vi "reset_channel.vi"(8 "error in (no error)":errorcluster, 10 "channel":T1=enum."1", 11 "Motech-pps-1200 in":refnum<class "Motech-pps-1200.lvclass">) -> (0 "error out":errorcluster, 3 "Motech-pps-1200 out":refnum<class "Motech-pps-1200.lvclass">)   [LabVIEW 2017, in "Motech-pps-1200.lvclass"]
uses:
  Motech-pps-1200.lvclass
  subVI/motech_power_supply/types/motech_set_value_cluster.ctl
  subVI/motech_power_supply/types/channels_enum.ctl
panel:
  in  "motech_set_value":T2={"voltage"=0.0, "current"=0.01, "channel"=enum."1"}
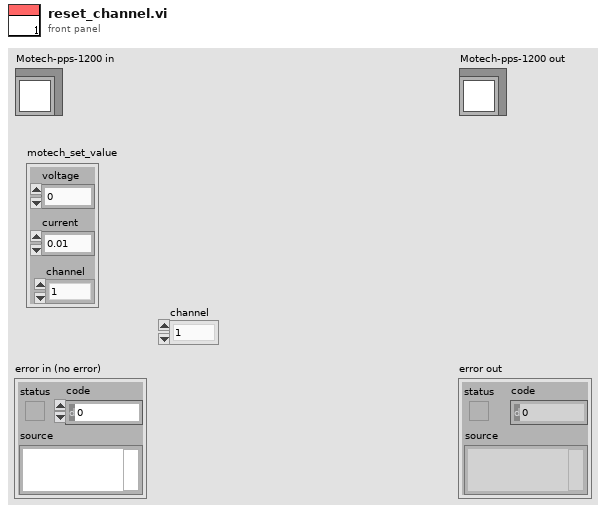
[diagram p1: front panel]
types:
  T1 = typedef "channels_enum.ctl" = enum16{"0", "1", "2"}
  T2 = typedef "motech_set_value_cluster.ctl" = cluster{"voltage":dbl, "current":dbl, "channel":T1}
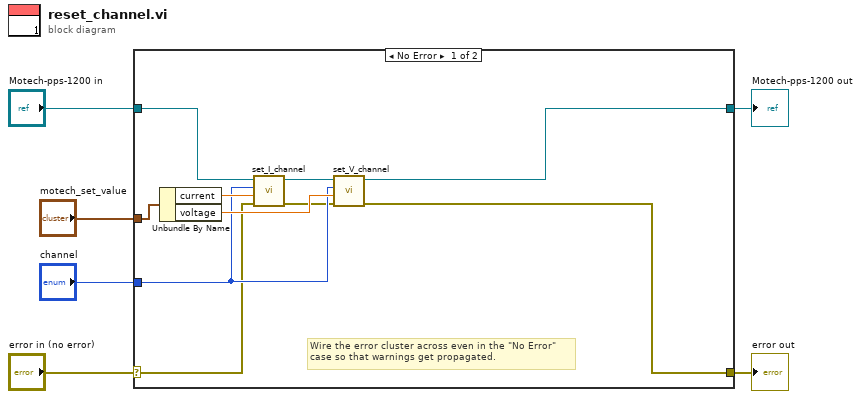
[diagram p0: block diagram]
diagram:
  n1 = case shown="No Error" "error in (no error)" {
    selector: "error in (no error)" -> [w9 w18]
    tunnel: [w7 w18] -> w5
    tunnel: [w14 w17] -> w3
    tunnel: "Motech-pps-1200 in" -> [w16 w17]
    tunnel: "motech_set_value" -> [w13 _]
    tunnel: "channel" -> [w10 _]
    frame No Error {
      # "Wire the error cluster across even in the \"No Error\"\ncase so that warnings get propagated."
      n2 = Unbundle By Name(w13) -> ("current"=w12:dbl, "voltage"=w11:dbl)
      n3 = call-dynamic "set_I_channel.vi"("error in (no error)"=w9, "current"=w12, "channel"=w10, "Motech-pps-1200 in"=w16) -> ("error out"=w8:errorcluster, "Motech-pps-1200 out"=w15:refnum<class "Motech-pps-1200.lvclass">)  [unwired: 6 in]
      n4 = call-dynamic "set_V_channel.vi"("error in (no error)"=w8, "voltage"=w11, "channel"=w10, "Motech-pps-1200 in"=w15) -> ("error out"=w7:errorcluster, "Motech-pps-1200 out"=w14:refnum<class "Motech-pps-1200.lvclass">)  [unwired: 6 in]
    }
    frame Error {
    }
  }
  "error out" <- w5
  "Motech-pps-1200 out" <- w3
